vi "(SubVI) Get TTB array from tick time.vi"(5 "Tick time (ms)":u32[](array[numeric])) -> (2 "TTB array (ms)\ntime axis (ms)":u32[](array[numeric]))   [LabVIEW 2014]
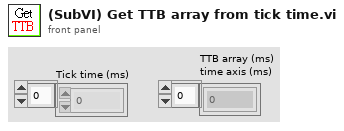
[diagram p1: front panel]
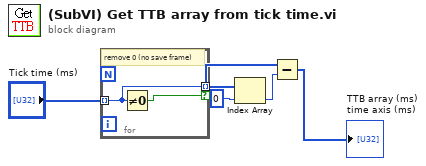
[diagram p0: block diagram]
diagram:
  n1 = for {
    tunnel: "Tick time (ms)" -> [w7] mode=indexing
    tunnel: [w7] -> w4 mode=indexing if=w6
    # "remove 0 (no save frame)"
    n2 = Not Equal To 0?(x=w7) -> (x != 0?=w6:bool)
  }
  n3 = Index Array(array=w4, index=0) -> (element=w1:u32)
  n4 = Subtract(x=w4, y=w1) -> (x-y=→"TTB array (ms)\ntime axis (ms)":u32[])
